vi "Encode Byte Array.vi"(10 "Array To Encode":u8[](array[numeric]), 11 "Image In":u8[](array[numeric])) -> (2 "Copies Encoded":i32, 3 "Image Out":u8[](array[numeric]))   [LabVIEW 2020]
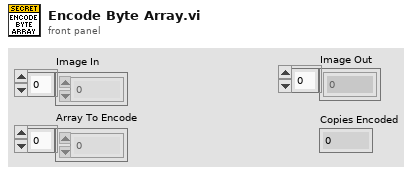
[diagram p1: front panel]
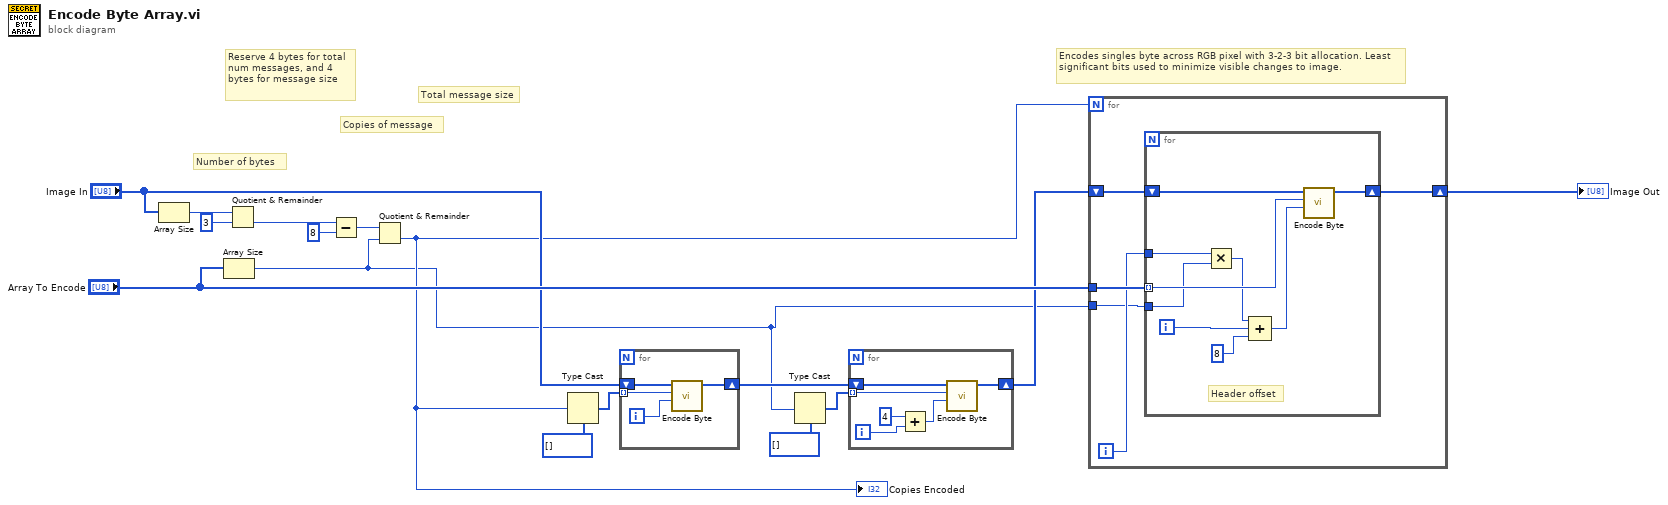
[diagram p0: block diagram]
diagram:
  # "Reserve 4 bytes for total num messages, and 4 bytes for message size"
  # "Encodes singles byte across RGB pixel with 3-2-3 bit allocation. Least significant bits used to minimize visible changes to image."
  # "Total message size"
  # "Copies of message"
  # "Number of bytes"
  n1 = Array Size(array="Image In") -> (size(s)=w16:i32)
  n2 = Array Size(array="Array To Encode") -> (size(s)=w1:i32)
  n3 = Quotient & Remainder(x=w16, y=3) -> (floor(x/y)=w12:i32)  [unwired: 1 out]
  n4 = Subtract(x=w12, y=8) -> (x-y=w10:i32)
  n5 = Quotient & Remainder(x=w10, y=w1) -> (floor(x/y)=w2:i32)  [unwired: 1 out]
  "Copies Encoded" <- w2
  n6 = Type Cast(type=u8[] [] ("Compressed Message 2"), x=w2) -> (*(type *) &x=w8:u8[])
  n7 = for {
    tunnel: w8 -> [w20] mode=indexing
    shift-right: [w17] -> w5
    shift-left: "Image In" -> [w18]
    i -> [w19]
    n8 = call "Encode Byte.vi"("Pixel Offset"=w19, "Byte To Encode"=w20, "Image In"=w18) -> ("Image Out"=w17:u8[])  [unwired: 8 in]
  }
  n9 = Type Cast(type=u8[] [] ("Compressed Message 2"), x=w1) -> (*(type *) &x=w7:u8[])
  n10 = for {
    tunnel: w7 -> [w26] mode=indexing
    shift-right: [w23] -> w3
    shift-left: w5 -> [w24]
    i -> [w25]
    n11 = Add(x=4 ("y"), y=w25) -> (x+y=w22:i32)
    n12 = call "Encode Byte.vi"("Pixel Offset"=w22, "Byte To Encode"=w26, "Image In"=w24) -> ("Image Out"=w23:u8[])  [unwired: 8 in]
  }
  n13 = for {
    N: w2 -> [_]
    tunnel: "Array To Encode" -> [w31]
    shift-right: [w30] -> w13
    shift-left: w3 -> [w29]
    tunnel: w1 -> [w27]
    i -> [w28]
    n14 = for {
      tunnel: w31 -> [w37] mode=indexing
      shift-right: [w35] -> w30
      shift-left: w29 -> [w38]
      tunnel: w28 -> [w34]
      tunnel: w27 -> [w33]
      i -> [w39]
      # "Header offset"
      n15 = Multiply(x=w34, y=w33) -> (x*y=w32:i32)
      n16 = Compound Arithmetic op=ADD(w32, w39, 8 ("y")) -> (w36:i32)
      n17 = call "Encode Byte.vi"("Pixel Offset"=w36, "Byte To Encode"=w37, "Image In"=w38) -> ("Image Out"=w35:u8[])  [unwired: 8 in]
    }
  }
  "Image Out" <- w13
